vi "Test Filter Dashed Class.vi"(8 "error in (no error)":errorcluster, 11 "Test Case In":refnum<class "Filter Test.lvclass">) -> (0 "error out":errorcluster, 3 "Test Case Out":refnum<class "Filter Test.lvclass">)   [LabVIEW 2020, in "Filter Test.lvclass"]
uses:
  Filter Test.lvclass
  C:/Program Files (x86)/National Instruments/LabVIEW 2020/vi.lib/Astemes/LUnit/Test Case.lvclass
  <vilib>/Astemes/LUnit/Test Case.lvclass/Test Case.ctl
  <vilib>/Astemes/LUnit/Append Pass Result.vi
  <vilib>/Astemes/LUnit/Append Fail Result.vi
  <vilib>/Astemes/LUnit/Describe Comparison.vi
  <vilib>/Astemes/LUnit/Compare Variants.vi
  <vilib>/Astemes/LUnit/Variant to string.vi
  <vilib>/Utility/Data Type/Get Type Information.vi
  <vilib>/Utility/LVClass/Get LV Class Name.vi
  source/Support/Filters/Dashed Filter/Dashed Filter.lvclass
  Filter Test.lvclass/Filter Test.ctl
  source/API/LUnit Test Suite/LUnit Test Suite.lvclass
  C:/Program Files (x86)/National Instruments/LabVIEW 2020/vi.lib/Astemes/LUnit/LUnit Runnable.lvclass
  C:/git/astemes-lunit/tests/Filter Test/Filter Test.lvclass
  <vilib>/Astemes/LUnit/Test Case.lvclass
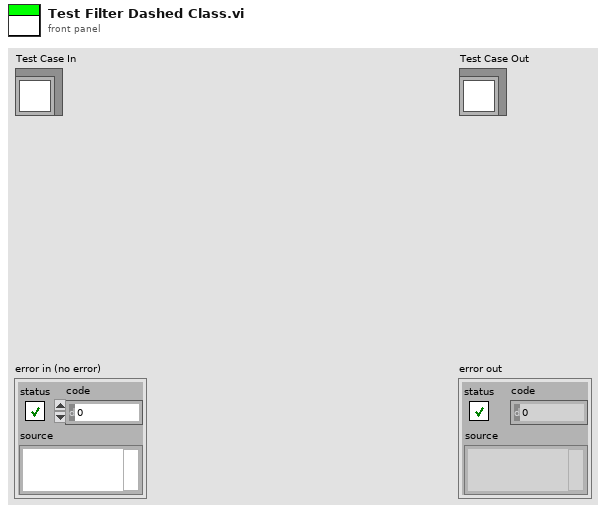
[diagram p1: front panel]
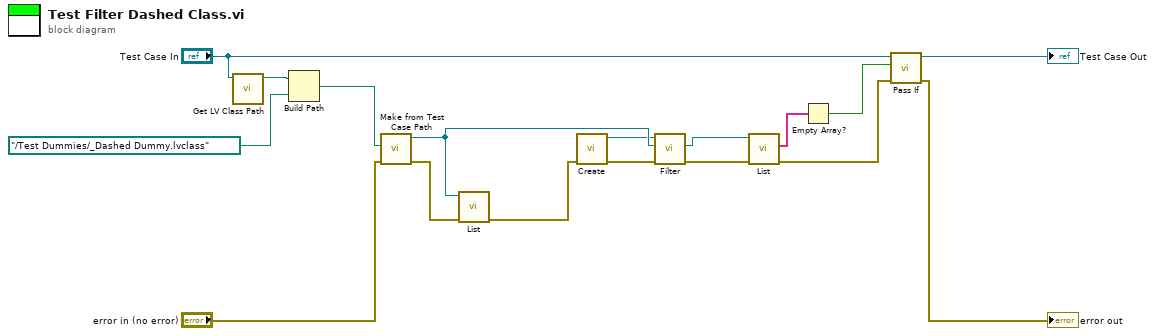
[diagram p0: block diagram]
diagram:
  n1 = call <vilib>:"Get LV Class Path.vi"("object"="Test Case In") -> ("class path"=w8:path)  [unwired: 9 in, 1 out]
  n2 = Build Path(base path=w8, name or relative path=path "../Test Dummies/_Dashed Dummy.lvclass") -> (appended path=w6:path)
  n3 = call "Make from Test Case Path.vi"("error in (no error)"="error in (no error)", "Test Case"=w6) -> ("error out"=w15:errorcluster, "LUnit Test Suite Out"=w10:refnum<class "LUnit Test Suite.lvclass">)  [unwired: 8 in]
  n4 = call "List.vi"("error in (no error)"=w15, "LUnit Test Suite In"=w10) -> ("error out"=w4:errorcluster)  [unwired: 8 in, 1 out]
  n5 = call "Create.vi"("error in (no error)"=w4) -> ("error out"=w3:errorcluster, "Dashed Filter"=w5:refnum<class "Dashed Filter.lvclass">)  [unwired: 9 in]
  n6 = call-dynamic "Filter.vi"("error in (no error)"=w3, "Test Suite"=w10, "Dashed Filter in"=w5) -> ("error out"=w13:errorcluster, "Filtered Test Suite"=w14:refnum<class "LUnit Test Suite.lvclass">)  [unwired: 7 in]
  n7 = call "List.vi"("error in (no error)"=w13, "LUnit Test Suite In"=w14) -> ("error out"=w12:errorcluster, "List of Runnables"=w2:string[])  [unwired: 8 in]
  n8 = Empty Array?(array=w2) -> (empty?=w1:bool)
  n9 = call <vilib>:"Pass If.vi"("error in (no error)"=w12, "Pass?"=w1, "LUnit Test Case In"="Test Case In") -> ("error out"=→"error out":errorcluster, "LUnit Test Case Out"=→"Test Case Out":refnum<class "Filter Test.lvclass">)  [unwired: 7 in]
